vi "EditorSub createPictureSub.vi"(8 "error in (no error)":errorcluster, 11 "XY Graph":refnum<vi>) -> (0 "error out":errorcluster, 3 "2D Picture":picture)   [LabVIEW 2018]
panel:
  out "tempGraph":cluster{"X":dbl[], "Y":sgl[]}[](graph)
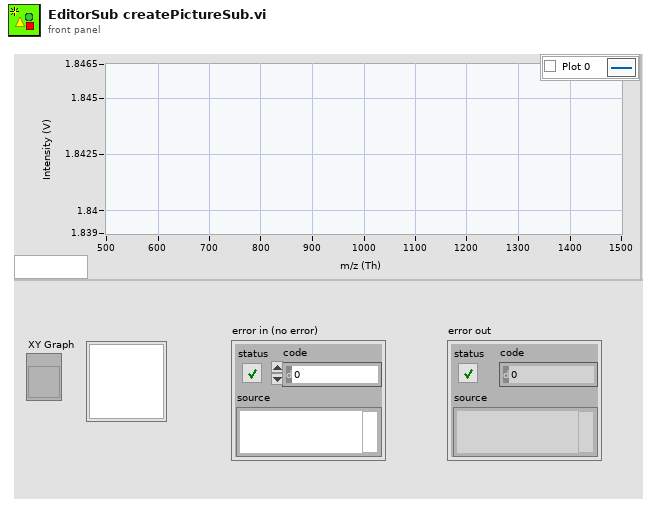
[diagram p1: front panel]
types:
  T1 = typedef "imagedata.ctl" = cluster{"image type":i32, "image depth":i32, "image":u8[], "mask":u8[], "colors":u32[], "Rectangle":cluster{"left":i16, "top":i16, "right":i16, "bottom":i16}}
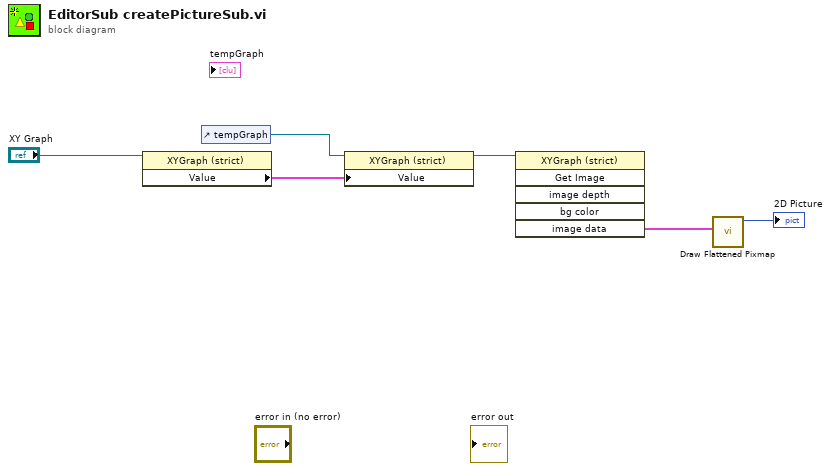
[diagram p0: block diagram]
diagram:
  n1 = property class="XYGraph (strict)"(reference="XY Graph") -> ("Value"=w4:cluster{"X":dbl[], "Y":sgl[]}[])  [unwired: 1 in, 2 out]
  n2 = control-ref of="tempGraph"() -> (w5:refnum<vi>)
  n3 = property class="XYGraph (strict)"(reference=w5, "Value"=w4) -> (reference out=w3:refnum<vi>)  [unwired: 1 in, 1 out]
  n4 = invoke class="XYGraph (strict)" method="Get Image"(reference=w3) -> ("image data"=w2:T1)  [unwired: 5 in, 5 out]
  n5 = call <vilib>:"Draw Flattened Pixmap.vi"("image data"=w2) -> ("new picture"=→"2D Picture":picture)  [unwired: 8 in]
